vi "Create Outline.vi"(5 "Bar Drawable":refnum<vi>, 7 "3D Bar Property":T1, 8 "error in (no error)":errorcluster, 10 "Plot Representation In":T3, 11 "Plot Object In":refnum<vi>) -> (0 "error out":errorcluster, 2 "Plot Representation Out":T3, 3 "Plot Object Out":refnum<vi>, 4 "Sector Object Out":refnum<vi>)   [LabVIEW 2017, in "3D Bar.lvclass"]
uses:
  <vilib>/Math Plots/3D Math Plots/3D Bar/3D Bar/3D Bar.lvclass
  <vilib>/Math Plots/3D Math Plots/3D Plot/3D Plot/Typedef/Plot Representation.ctl
  <vilib>/Math Plots/3D Math Plots/3D Plot/3D Plot/Typedef/Range Clusters.ctl
  <vilib>/Math Plots/3D Math Plots/3D Plot/3D Plot/Typedef/Mesh Data.ctl
  <vilib>/Math Plots/3D Math Plots/3D Bar/3D Bar/Typedef/3D Bar Property.ctl
  <vilib>/Math Plots/3D Math Plots/3D Plot/3D Plot/Typedef/Line Type.ctl
  <vilib>/picture/3D Picture Control/Object/Create Object (name).vi
  <vilib>/picture/3D Picture Control/NI_3D Picture Control.lvlib
  <vilib>/Math Plots/3D Math Plots/3D Plot/3D Plot/3D Plot.lvclass
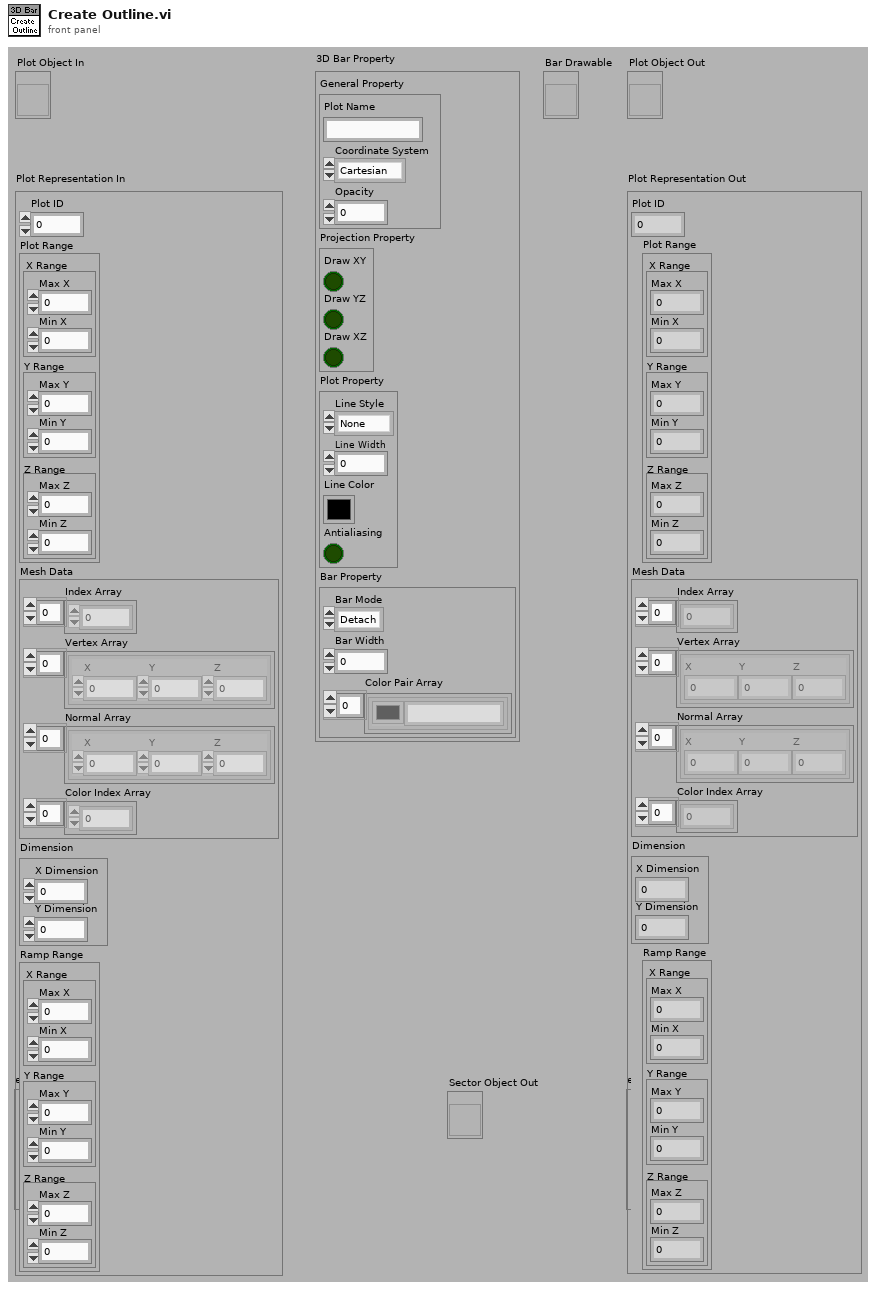
[diagram p1: front panel]
types:
  T1 = typedef "3D Bar.lvclass/3D Bar Property.ctl" = cluster{"General Property":cluster{"Plot Name":string, "Coordinate System":enum16{"Cartesian", "Cylindrical", "Spherical"}, "Opacity":sgl}, "Projection Property":cluster{"Draw XY":bool, "Draw YZ":bool, "Draw XZ":bool}, "Plot Property":cluster{"Line Style":T2, "Line Width":sgl, "Line Color":u32, "Antialiasing":bool}, "Bar Property":cluster{"Bar Mode":enum16{"Detach", "Group", "Stack"}, "Bar Width":sgl, "Color Pair Array":cluster{"Color":u32, "String":string}[]}}
  T2 = typedef "3D Plot.lvclass/Line Type.ctl" = enum16{"None", "Solid", "Dash", "Dot", "Dash Dot"}
  T3 = typedef "3D Plot.lvclass/Plot Representation.ctl" = cluster{"Plot ID":i32, "Plot Range":T4, "Mesh Data":T5, "Dimension":cluster{"X Dimension":i32, "Y Dimension":i32}, "Ramp Range":T4}
  T4 = typedef "3D Plot.lvclass/Range Clusters.ctl" = cluster{"X Range":cluster{"Max X":sgl, "Min X":sgl}, "Y Range":cluster{"Max Y":sgl, "Min Y":sgl}, "Z Range":cluster{"Max Z":sgl, "Min Z":sgl}}
  T5 = typedef "3D Plot.lvclass/Mesh Data.ctl" = cluster{"Index Array":u32[], "Vertex Array":cluster{"X":sgl, "Y":sgl, "Z":sgl}[], "Normal Array":cluster{"X":sgl, "Y":sgl, "Z":sgl}[], "Color Index Array":i32[]}
  T6 = enum16{"Points", "Lines", "Line Strip", "Line Loop", "Triangles", "Triangle Strip", "Triangle Fan", "Quads", "Quad Strip", "Polygon"}
  T7 = enum16{"Overall", "Per Primitive", "Per Vertex", "Binding Off"}
  T8 = enum16{"Inherit Value", "Points", "Wireframe", "Polygons"}
  T9 = enum16{"Normal Bin", "Opaque Bin", "Transparent Bin"}
  T10 = enum16{"Inherit Material", "Use entire Material", "Ignore Ambient", "Ignore Diffuse", "Ignore Specular", "Ignore Emission", "Ignore Ambient and Diffuse"}
  T11 = enum16{"Inherit Value", "Counterclockwise", "Clockwise"}
  T12 = typedef "LV3DPointTypeDef.ctl" = cluster{"X":sgl, "Y":sgl, "Z":sgl}
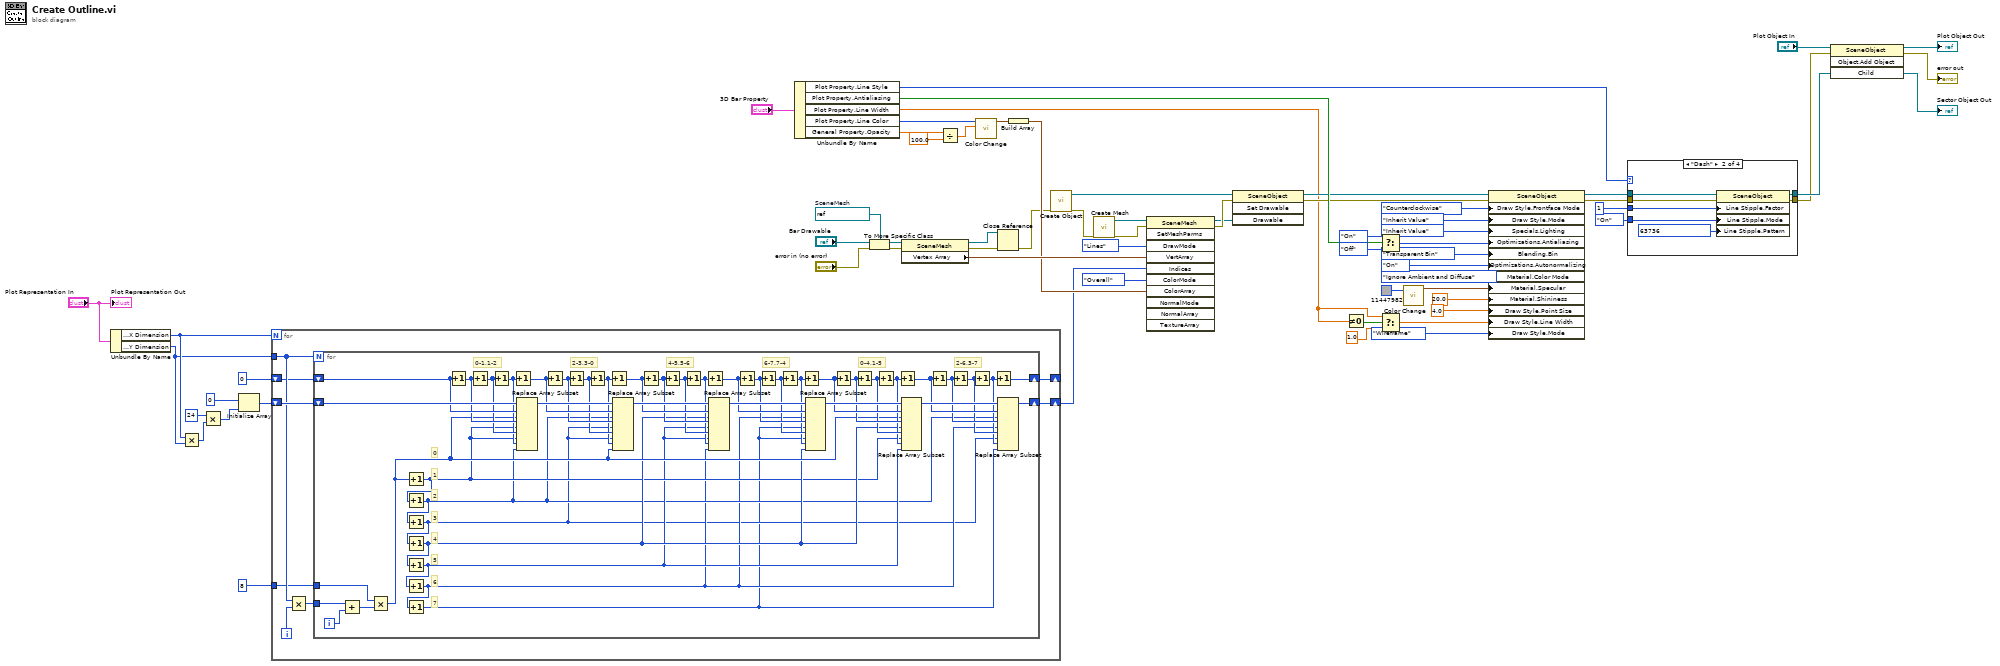
[diagram p0: block diagram]
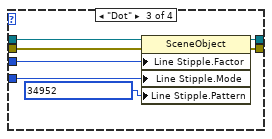
[diagram p3: hidden frame]
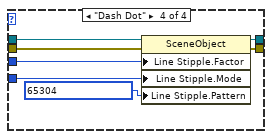
[diagram p4: hidden frame]
diagram:
  w32 = refnum<vi> refnum  # SceneMesh
  n1 = Unbundle By Name("Plot Representation In") -> ("Dimension.X Dimension"=w10:i32, "Dimension.Y Dimension"=w9:i32)
  n2 = Multiply(x=w10, y=w9) -> (x*y=w16:i32)
  n3 = Multiply(x=24 ("value"), y=w16) -> (x*y=w12:i32)
  n4 = Initialize Array(u32 0 ("value"), w12) -> (w13:u32[])
  n5 = for {
    N: w10 -> [_]
    shift-right: [w74] -> w7
    shift-left: w13 -> [w75]
    tunnel: w9 -> [w71]
    tunnel: 8 ("value") -> [w70]
    shift-right: [w68] -> _
    shift-left: 0 ("value") -> [w69]
    i -> [w73]
    n6 = Multiply(x=w71, y=w73) -> (x*y=w72:i32)
    n7 = for {
      N: w71 -> [_]
      shift-right: [w109] -> w74
      shift-left: w75 -> [w115]
      tunnel: w72 -> [w119]
      tunnel: w70 -> [w116]
      shift-right: [w108] -> w68
      shift-left: w69 -> [w107]
      i -> [w118]
      # "2-6,3-7"
      # "0-4,1-5"
      # "6-7,7-4"
      # "4-5,5-6"
      # "2-3,3-0"
      # "0-1,1-2"
      # "7"
      # "6"
      # "5"
      # "4"
      # "3"
      # "2"
      # "1"
      # "0"
      n8 = Add(x=w119, y=w118) -> (x+y=w117:i32)
      n9 = Multiply(x=w116, y=w117) -> (x*y=w83:i32)
      n10 = Increment(x=w83) -> (x+1=w81:i32)
      n11 = Increment(x=w81) -> (x+1=w79:i32)
      n12 = Increment(x=w79) -> (x+1=w77:i32)
      n13 = Increment(x=w77) -> (x+1=w82:i32)
      n14 = Increment(x=w82) -> (x+1=w80:i32)
      n15 = Increment(x=w80) -> (x+1=w78:i32)
      n16 = Increment(x=w78) -> (x+1=w76:i32)
      n17 = Increment(x=w107) -> (x+1=w106:i32)
      n18 = Increment(x=w106) -> (x+1=w105:i32)
      n19 = Increment(x=w105) -> (x+1=w104:i32)
      n20 = Increment(x=w104) -> (x+1=w103:i32)
      n21 = Replace Array Subset(array=w115, new element #1=w83, index #1=w107, new element #2=w81, index #2=w106, new element #3=w81, index #3=w105, new element #4=w79, index #4=w104) -> (w114:u32[])
      n22 = Increment(x=w103) -> (x+1=w102:i32)
      n23 = Increment(x=w102) -> (x+1=w101:i32)
      n24 = Increment(x=w101) -> (x+1=w100:i32)
      n25 = Increment(x=w100) -> (x+1=w99:i32)
      n26 = Replace Array Subset(array=w114, new element #1=w79, index #1=w103, new element #2=w77, index #2=w102, new element #3=w77, index #3=w101, new element #4=w83, index #4=w100) -> (w113:u32[])
      n27 = Increment(x=w99) -> (x+1=w98:i32)
      n28 = Increment(x=w98) -> (x+1=w97:i32)
      n29 = Increment(x=w97) -> (x+1=w96:i32)
      n30 = Increment(x=w96) -> (x+1=w95:i32)
      n31 = Replace Array Subset(array=w113, new element #1=w82, index #1=w99, new element #2=w80, index #2=w98, new element #3=w80, index #3=w97, new element #4=w78, index #4=w96) -> (w112:u32[])
      n32 = Increment(x=w95) -> (x+1=w94:i32)
      n33 = Increment(x=w94) -> (x+1=w93:i32)
      n34 = Increment(x=w93) -> (x+1=w92:i32)
      n35 = Increment(x=w92) -> (x+1=w91:i32)
      n36 = Replace Array Subset(array=w112, new element #1=w78, index #1=w95, new element #2=w76, index #2=w94, new element #3=w76, index #3=w93, new element #4=w82, index #4=w92) -> (w111:u32[])
      n37 = Increment(x=w91) -> (x+1=w90:i32)
      n38 = Increment(x=w90) -> (x+1=w89:i32)
      n39 = Increment(x=w89) -> (x+1=w88:i32)
      n40 = Increment(x=w88) -> (x+1=w87:i32)
      n41 = Replace Array Subset(array=w111, new element #1=w83, index #1=w91, new element #2=w82, index #2=w90, new element #3=w81, index #3=w89, new element #4=w80, index #4=w88) -> (w110:u32[])
      n42 = Increment(x=w87) -> (x+1=w86:i32)
      n43 = Increment(x=w86) -> (x+1=w85:i32)
      n44 = Increment(x=w85) -> (x+1=w84:i32)
      n45 = Increment(x=w84) -> (x+1=w108:i32)
      n46 = Replace Array Subset(array=w110, new element #1=w79, index #1=w87, new element #2=w78, index #2=w86, new element #3=w77, index #3=w85, new element #4=w76, index #4=w84) -> (w109:u32[])
    }
  }
  n47 = Unbundle By Name("3D Bar Property") -> ("Plot Property.Line Style"=w34:T2, "Plot Property.Antialiasing"=w50:bool, "Plot Property.Line Width"=w1:sgl, "Plot Property.Line Color"=w47:u32, "General Property.Opacity"=w46:sgl)
  n48 = To More Specific Class(target class=w32, reference="Bar Drawable", error in="error in (no error)") -> (specific class reference=w31:refnum<vi>, error out=w19:errorcluster)
  n49 = property class="SceneMesh"(reference=w31, error in=w19) -> (reference out=w4:refnum<vi>, error out=w3:errorcluster, "Vertex Array"=w23:T12[])
  n50 = Divide(x=w46, y=sgl 100.0) -> (x/y=w42:sgl)
  n51 = call <vilib>:"Color Change.vi"("Alpha"=w42, "Color"=w47) -> ("RGBA"=w33:cluster{"R":sgl, "G":sgl, "B":sgl, "A":sgl})  [unwired: 9 out]
  n52 = Close Reference(reference=w4, error in (no error)=w3) -> (error out=w2:errorcluster)
  n53 = Build Array(w33) -> (w22:cluster{"R":sgl, "G":sgl, "B":sgl, "A":sgl}[])
  n54 = call-poly <vilib>:"Create Object.vi"("error in (no error)"=w2) -> ("error out"=w24:errorcluster, "Scene:New Object"=w25:refnum<vi>)  [unwired: 9 in]
  n55 = call <vilib>:"Create Mesh.vi"("error in (no error)"=w24) -> ("error out"=w29:errorcluster, "New Mesh Refnum"=w26:refnum<vi>)  [unwired: 9 in]
  n56 = invoke class="SceneMesh" method="SetMeshParms"(reference=w26, error in=w29, "DrawMode"=T6."Lines" ("Draw Mode"), "VertArray"=w23, "Indices"=w7, "ColorMode"=T7."Overall" ("Color Binding Mode"), "ColorArray"=w22) -> (reference out=w27:refnum<vi>, error out=w28:errorcluster)  [unwired: 4 in, 9 out]
  n57 = invoke class="SceneObject" method="Set Drawable"(reference=w25, error in=w28, "Drawable"=w27) -> (reference out=w21:refnum<vi>, error out=w20:errorcluster)  [unwired: 1 in, 2 out]
  n58 = Not Equal To 0?(x=w1) -> (x != 0?=w45:bool)
  n59 = Select(t=enum16{"Inherit Value", "Off", "On"}."On" ("Specials:Antialiasing"), s=w50, f=enum16{"Inherit Value", "Off", "On"}."Off") -> (s? t:f=w49:enum16{"Inherit Value", "Off", "On"})
  n60 = Select(t=w1, s=w45, f=sgl 1.0) -> (s? t:f=w43:sgl)
  n61 = call <vilib>:"Color Change.vi"("Color"=u32 11447982) -> ("RGBA"=w59:cluster{"R":sgl, "G":sgl, "B":sgl, "A":sgl})  [unwired: 1 in, 9 out]
  n62 = property class="SceneObject"(reference=w21, error in=w20, "Draw Style.Frontface Mode"=T11."Counterclockwise" ("Draw Style:Frontface Mode"), "Draw Style.Mode"=T8."Inherit Value" ("Draw Style:Mode"), "Specials.Lighting"=enum16{"Inherit Value", "Off", "On"}."Inherit Value" ("Specials:Lighting"), "Optimizations.Antialiasing"=w49, "Blending.Bin"=T9."Transparent Bin" ("Blending:Bin"), "Optimizations.Autonormalizing"=enum16{"Inherit Value", "Off", "On"}."On" ("Optimizations:Autonormalizing"), "Material.Color Mode"=T10."Ignore Ambient and Diffuse" ("Material:Color Mode"), "Material.Specular"=w59, "Material.Shininess"=sgl 20.0 ("Material:Shininess"), "Draw Style.Point Size"=sgl 4.0 ("Draw Style:Point Size"), "Draw Style.Line Width"=w43, "Draw Style.Mode"=T8."Wireframe" ("Draw Style:Mode")) -> (reference out=w40:refnum<vi>, error out=w39:errorcluster)
  n63 = case shown="\"Dash\"" w34 {
    tunnel: w40 -> [w121 w128 w135 w142]
    tunnel: [w121 w127 w131 w138] -> w36
    tunnel: w39 -> [w120 w126 w134 w141]
    tunnel: [w120 w125 w130 w137] -> w35
    tunnel: enum16{"Inherit Value", "Off", "On"}."On" ("Line Stipple:Mode") -> [_ w124 w132 w139]
    tunnel: 1 ("Line Stipple:Factor") -> [_ w123 w133 w140]
    frame "Solid", Default {
    }
    frame "Dash" {
      n64 = property class="SceneObject"(reference=w128, error in=w126, "Line Stipple.Factor"=w123, "Line Stipple.Mode"=w124, "Line Stipple.Pattern"=u16 63736 ("Line Stipple:Factor")) -> (reference out=w127:refnum<vi>, error out=w125:errorcluster)
    }
    frame "Dot" {
      n65 = property class="SceneObject"(reference=w135, error in=w134, "Line Stipple.Factor"=w133, "Line Stipple.Mode"=w132, "Line Stipple.Pattern"=u16 34952 ("Line Stipple:Factor")) -> (reference out=w131:refnum<vi>, error out=w130:errorcluster)
    }
    frame "Dash Dot" {
      n66 = property class="SceneObject"(reference=w142, error in=w141, "Line Stipple.Factor"=w140, "Line Stipple.Mode"=w139, "Line Stipple.Pattern"=u16 65304 ("Line Stipple:Factor")) -> (reference out=w138:refnum<vi>, error out=w137:errorcluster)
    }
  }
  n67 = invoke class="SceneObject" method="Object.Add Object"(reference="Plot Object In", error in=w35, "Child"=w36) -> (reference out=→"Plot Object Out":refnum<vi>, error out=→"error out":errorcluster, "Child"=→"Sector Object Out":refnum<vi>)  [unwired: 1 in, 1 out]
  "Plot Representation Out" <- "Plot Representation In"
